vi "ctrlHeadingOnWP-DP.vi"(1 "p(t)":dbl[](array[numeric]), 2 "psi":dbl, 3 "p_d":dbl[](array[numeric])) -> (9 "psiplot":cluster{"Double":dbl, "y_r":dbl, "y":dbl}, 11 "yplot":cluster{"Double":dbl, "y_r":dbl, "y":dbl}, 13 "xplot":cluster{"Double":dbl, "y_r":dbl, "y":dbl}, 15 "U":dbl[](array[numeric]), 17 "eta_e_n":dbl[](array[numeric]), 18 "eta_e_b":dbl[](array[numeric]))   [LabVIEW 2014]
uses:
  <vilib>/Simulation/Scripting/Companion Diagram/SimConfigNode/SimParams.ctl
  <vilib>/Simulation/Scripting/Companion Diagram/SimConfigNode/_simSolvers.ctl
  <vilib>/Simulation/Implementation/Shared/SIMSCR Execution Mode.ctl
  <vilib>/Simulation/Param Hierarchy/Typedefs/SIMPH Param Control Actions.ctl
  <vilib>/Simulation/Implementation/Shared/NILVSim_ParamChanged.vi
  <vilib>/Simulation/Implementation/Shared/NILVSIM_BeginStep.vi
  <vilib>/Simulation/Implementation/Shared/NILVSim_Manager.vi
  <vilib>/Utility/error.llb/Clear Errors.vi
  <vilib>/Simulation/Implementation/Shared/NILVSim_FinalizeModel.vi
  <vilib>/Simulation/Implementation/Shared/SIM Unbundle Sim Info.vi
  <vilib>/Simulation/Implementation/Shared/NILVSim_Initialize.vi
  <vilib>/Simulation/Utility/Implementation/NILVSim Get Time and IsAcceptedStep.vi
  <vilib>/Simulation/Implementation/Shared/SIMSH Read Queue.vi
  <vilib>/Simulation/Implementation/Shared/NILVSim_GetModelError.vi
  <vilib>/Simulation/Implementation/Shared/SIM Bundle Sim Info.vi
  <vilib>/imath/engines/lvmath2/RunTimeEngine/NodeEndStatement/NIMS_NodeEndStatement_Output.vi
  <instcachedir>/0/NIMS_NodeEndStatement_Output_53EC0D466D134D7ABD903AC30B43404B.lvgen/NIMS_NodeEndStatement_Output_53EC0D466D134D7ABD903AC30B43404B_001.vi
  <vilib>/imath/engines/lvmath2/RunTimeEngine/ErrorHandling/NIMS_Finalize Error.vi
  <vilib>/addons/control/pid/pid.llb/PID (DBL).vi
  <vilib>/Simulation/Implementation/XNodeFramework/SimXNode/SimX.xnode
  subVIs/refModelDP3rd.vi
  <vilib>/Simulation/Scripting/Companion Diagram/SimConfigNode/SimDog.xnode
  <vilib>/addons/control/pid/NI_PID_pid.lvlib
  <vilib>/Simulation/Implementation/Shared/NI_SIM_Implementation.lvlib
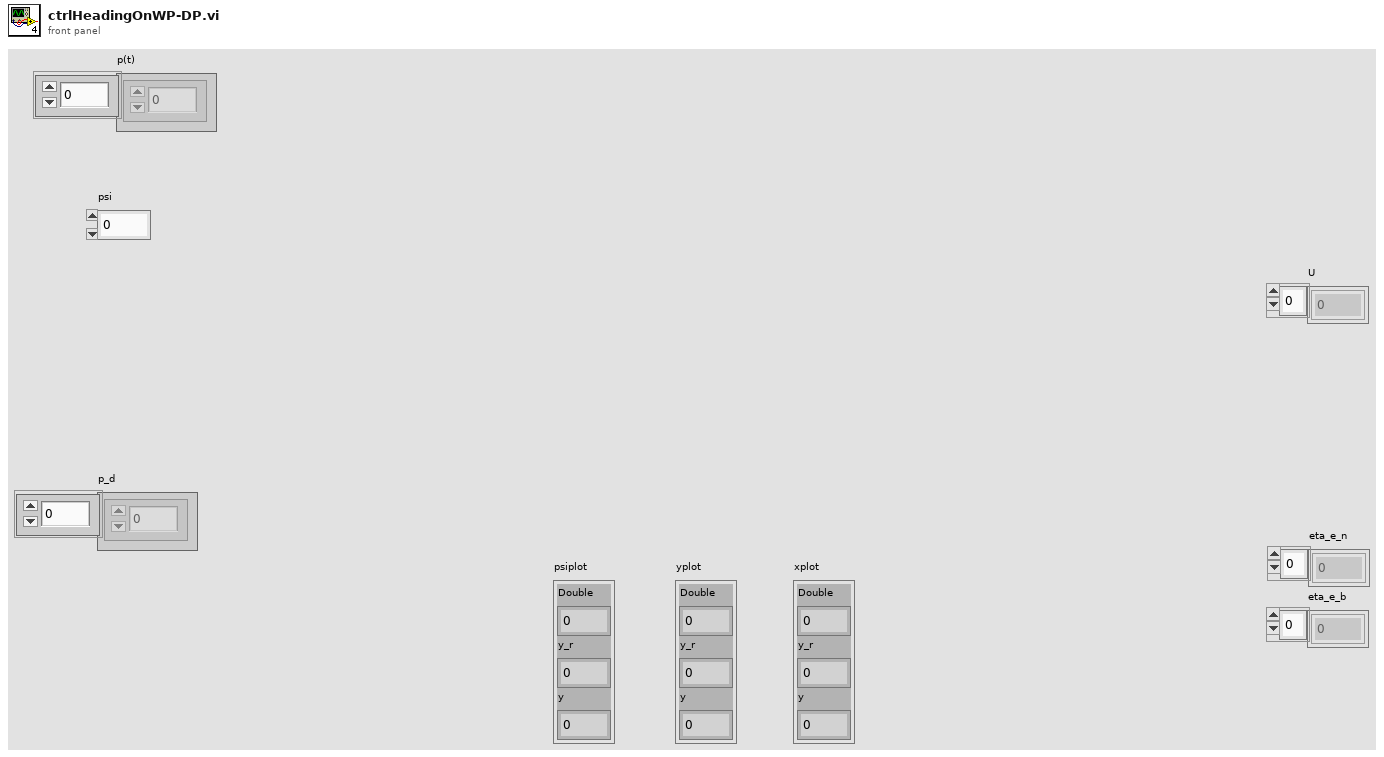
[diagram p1: front panel]
types:
  T1 = cluster{"proportional gain (Kc)":dbl, "integral time (Ti, min)":dbl, "derivative time (Td, min)":dbl}
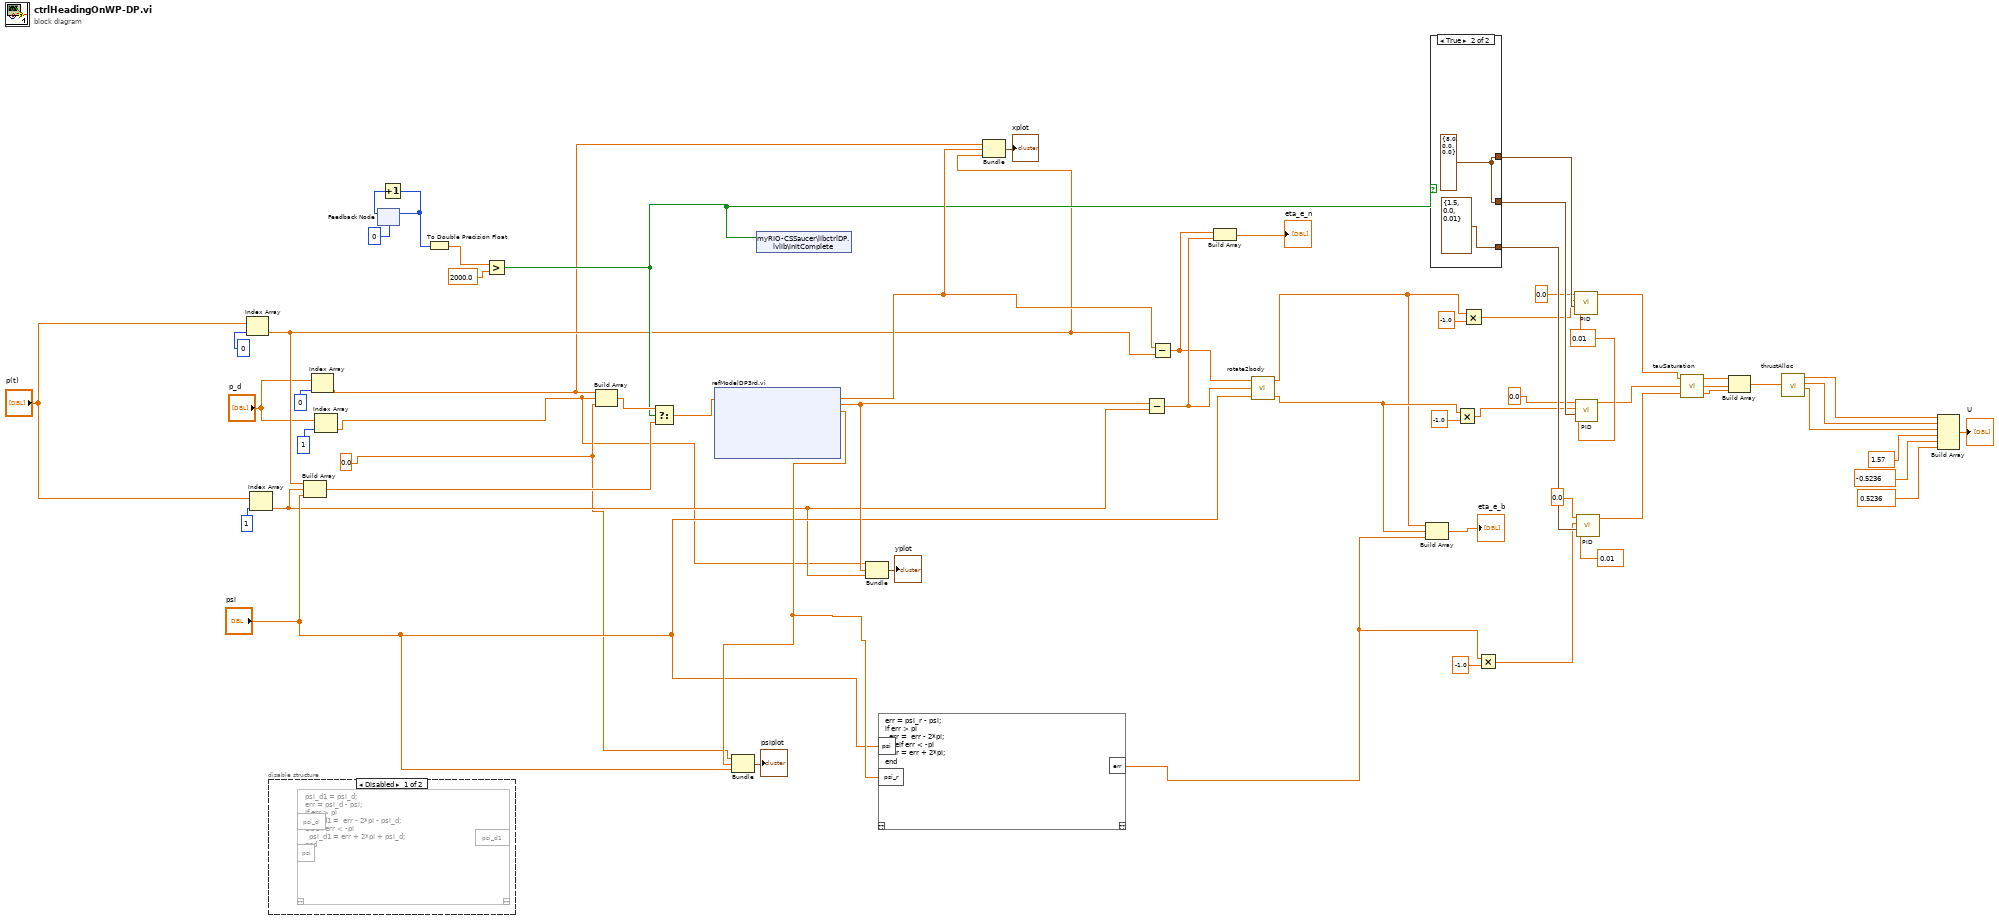
[diagram p0: block diagram]
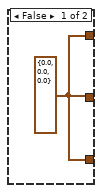
[diagram p3: hidden frame]
diagram:
  w6 = 0.0
  w62 = 0.01 ("dt (s)")
  n1 = Index Array(array="p(t)", index=0) -> (element=w18:dbl)
  n2 = Index Array(array="p(t)", index=1) -> (element=w16:dbl)
  n3 = disable-structure shown="Disabled" {
    frame Disabled {
      n4 = mathscript code="psi_d1 = psi_d;\nerr = psi_d - psi;\nif err > pi\n  psi_d1 =  err - 2*pi - psi_d;\nelseif err < -pi\n  psi_d1 = err + 2*pi + psi_d;\nend"() -> ()  [unwired: 3 in, 2 out]
    }
    frame Enabled {
    }
  }
  n5 = Build Array(w18, w16, "psi") -> (w28:dbl[])
  n6 = Index Array(array="p_d", index=0) -> (element=w3:dbl)
  n7 = Index Array(array="p_d", index=1) -> (element=w4:dbl)
  n8 = feedback #1(u32 0 ("f")) -> (w24:u32)
  n9 = Increment(x=w24) -> (x+1=w22:u32)
  n10 = feedback-in #1(w22) -> ()
  n11 = To Double Precision Float(number=w22) -> (double precision float=w23:dbl)
  n12 = Greater?(x=w23, y=2000.0) -> (0:w26:bool)
  n13 = Build Array(w3, w4, w6) -> (w29:dbl[])
  n14 = Select(t=w29, s=w26, f=w28) -> (s? t:f=w27:dbl[])
  n15 = xnode "refModelDP3rd.vi"("eta_d"=w27) -> ("x_r"=w38:dbl, "y_r"=w37:dbl, "psi_r"=w21:dbl)  [unwired: 2 in, 9 out]
  n16 = Bundle(w6, "psi_r"=w21, "psi"="psi") -> (→"psiplot":cluster{dbl, "psi_r":dbl, "psi":dbl})  [unwired: 1 in]
  n17 = shared-variable "myRIO-CSSaucer\\libctrlDP.lvlib\\initComplete"(w26) -> ()  [unwired: 1 in, 1 out]
  n18 = Bundle("y"=w4, "y_r"=w37, "y"=w16) -> (→"yplot":cluster{"y":dbl, "y_r":dbl, "y":dbl})  [unwired: 1 in]
  n19 = mathscript code="err = psi_r - psi;\nif err > pi\n  err =  err - 2*pi;\nelseif err < -pi\n  err = err + 2*pi;\nend"("psi"="psi", "psi_r"=w21) -> ("err"=w20:dbl)  [unwired: 1 in, 1 out]
  n20 = Bundle("y"=w3, "x_r"=w38, "y"=w18) -> (→"xplot":cluster{"y":dbl, "x_r":dbl, "y":dbl})  [unwired: 1 in]
  n21 = Subtract(x=w37, y=w16) -> (x-y=w55:dbl)
  n22 = Subtract(x=w38, y=w18) -> (x-y=w54:dbl)
  n23 = Build Array(w54, w55) -> (→"eta_e_n":dbl[])
  n24 = call "rotate2body.vi"("psi"="psi", "2"=w55, "1"=w54) -> ("2_body"=w48:dbl, "1_body"=w43:dbl)  [unwired: 1 in]
  n25 = Build Array(w43, w48, w20) -> (→"eta_e_b":dbl[])
  n26 = case shown="True" w26 {
    tunnel: [w141 w142] -> w59
    tunnel: [w141 w142] -> w58
    tunnel: [w141 T1 {"proportional gain (Kc)"=1.5, "integral time (Ti, min)"=0.0, "derivative time (Td, min)"=0.01} ("PID 0")] -> w57
    frame False {
      w141 = T1 {"proportional gain (Kc)"=0.0, "integral time (Ti, min)"=0.0, "derivative time (Td, min)"=0.0} ("PID 0")
    }
    frame True {
      w142 = T1 {"proportional gain (Kc)"=8.0, "integral time (Ti, min)"=0.0, "derivative time (Td, min)"=0.0} ("PID 0")
    }
  }
  n27 = Multiply(x=w48, y=-1.0) -> (x*y=w47:dbl)
  n28 = Multiply(x=w43, y=-1.0) -> (x*y=w41:dbl)
  n29 = Multiply(x=w20, y=-1.0) -> (x*y=w39:dbl)
  n30 = call-poly <vilib>:"PID.vi"("dt (s)"=w62, "PID gains"=w59, "process variable"=w41, "setpoint"=0.0 ("process variable")) -> ("output"=w34:dbl)  [unwired: 6 in, 1 out]
  n31 = call-poly <vilib>:"PID.vi"("dt (s)"=w62, "PID gains"=w58, "process variable"=w47, "setpoint"=0.0 ("process variable")) -> ("output"=w35:dbl)  [unwired: 6 in, 1 out]
  n32 = call-poly <vilib>:"PID.vi"("dt (s)"=0.01, "PID gains"=w57, "process variable"=w39, "setpoint"=0.0 ("process variable")) -> ("output"=w36:dbl)  [unwired: 6 in, 1 out]
  n33 = call "tauSaturation.vi"("N"=w36, "Y"=w35, "X"=w34) -> ("Nout"=w31:dbl, "Yout"=w32:dbl, "Xout"=w33:dbl)
  n34 = Build Array(w33, w32, w31) -> (w60:dbl[])
  n35 = call "thrustAlloc.vi"("tau"=w60) -> ("u_0"=w8:dbl, "u_1"=w9:dbl, "u_2"=w10:dbl)  [unwired: 5 in]
  n36 = Build Array(w8, w9, w10, 1.57 ("element"), -0.5236 ("element"), 0.5236 ("element")) -> (→"U":dbl[])
